vi "Actor Core.vi"(8 "error in":errorcluster, 11 "My Application":refnum<class "UI.lvclass">) -> (0 "error out":errorcluster, 3 "Actor out":refnum<class "Actor.lvclass">)   [LabVIEW 2025, in "UI.lvlib" / "UI.lvclass"]
doc: "This is Actor Core.vi, the main message handling loop for Actors. An actor usually just sits in this loop and processes messages as they arrive. Any error returned by the message Do.vi call will stop the loop, with error code 43 as the canonical signal to stop with no error sent to caller. Descendants may override that in Handle Error.vi."
uses:
  UI.lvclass
  C:/Program Files (x86)/National Instruments/LabVIEW 2025/vi.lib/ActorFramework/Actor/Actor.lvclass
  <vilib>/ActorFramework/Actor/Actor.lvclass
  Geocoding Actor/Geocoding/Country.ctl
  Geocoding Actor/Geocoding/Geocoding.lvclass
  Weather Actor/Weather/Weather.lvclass
  Geocoding Actor/Geocoding/Geocoding.lvclass/Geocoding.ctl
  Weather Actor/Weather/Weather.lvclass/Weather.ctl
  UI.lvclass/UI.ctl
  <vilib>/ActorFramework/Actor/Actor.lvclass/Actor.ctl
  <vilib>/ActorFramework/Message Enqueuer/Message Enqueuer.lvclass/Message Enqueuer.ctl
  Geocoding Actor/Geocoding Messages/Get Geo Codes Msg/Get Geo Codes Msg.lvclass/Get Geo Codes Msg.ctl
  Weather Actor/Weather Messages/Get Weather Forecast Data Msg/Get Weather Forecast Data Msg.lvclass/Get Weather Forecast Data Msg.ctl
  <vilib>/ActorFramework/Message Enqueuer/Init from Existing Queue.vi
  <vilib>/ActorFramework/Message Enqueuer/Enqueue.vi
  <vilib>/ActorFramework/Stop Msg/Stop Msg.lvclass
  C:/Program Files (x86)/National Instruments/LabVIEW 2025/vi.lib/ActorFramework/Message/Message.lvclass
  Geocoding Actor/Geocoding Messages/Get Geo Codes Msg/Get Geo Codes Msg.lvclass
  Weather Actor/Weather Messages/Get Weather Forecast Data Msg/Get Weather Forecast Data Msg.lvclass
  <vilib>/ActorFramework/Message Priority Queue/Priority Enqueue.vi
  <vilib>/ActorFramework/Message Enqueuer/Message Enqueuer.lvclass
panel:
  out "Results":T1(array[cluster])
  out "Weather Forecast Data":T2(graph)
  in  "Country":T3=enum."Germany"
  in  "City":string
  out "Table Control":string[][](table)
  in  "stop signal":bool
  in  "Stop":bool
  in  "Get City Data":bool
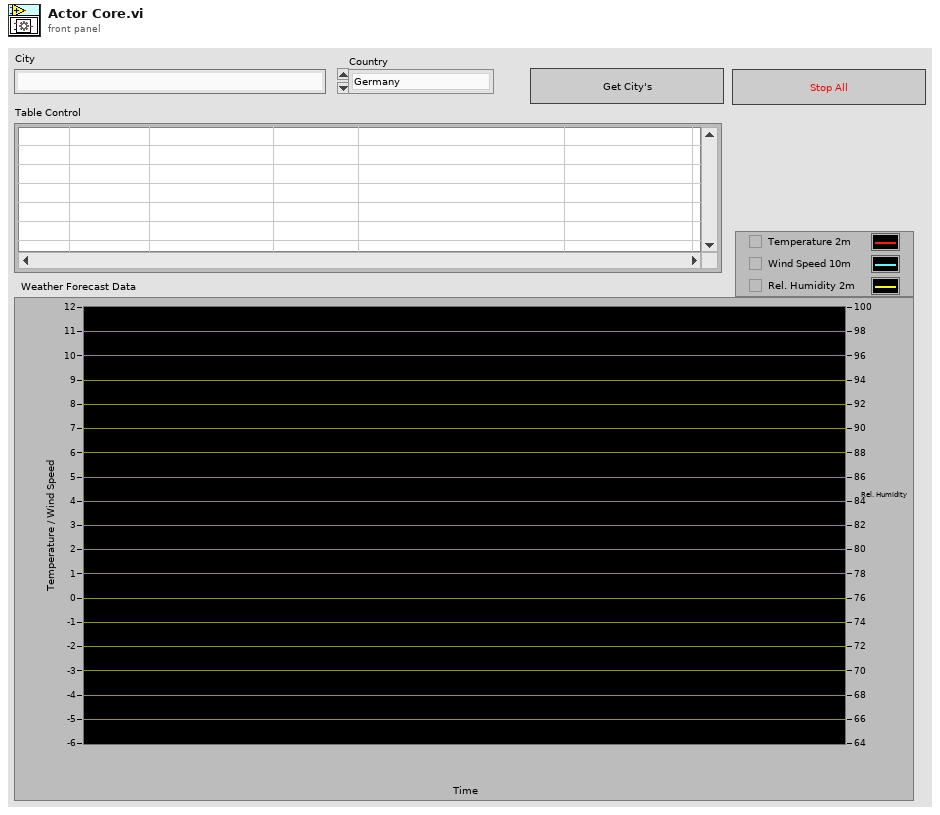
[diagram p1: front panel]
types:
  T1 = cluster{"id":i32, "name":string, "latitude":dbl, "longitude":dbl, "elevation":dbl, "feature_code":string, "country_code":string, "timezone":string, "population":i32, "postcodes":string[], "admin1":string, "admin2":string, "admin3":string, "admin4":string, "admin1_id":i32, "admin2_id":i32, "admin3_id":i32, "admin4_id":i32}[]
  T2 = cluster{timestamp[], "relative_humidity_2m":dbl[]}[]
  T3 = typedef "Geocoding Actor.lvlib/Geocoding.lvclass/Country.ctl" = enum16{"Austria", "Germany", "Switzerland"}
  T4 = typedef "LVRowAndColumnTypeDef.ctl" = cluster{"Row":i32, "Column":i32}
  T5 = cluster{"id":i32, "name":string, "latitude":dbl, "longitude":dbl, "elevation":dbl, "feature_code":string, "country_code":string, "timezone":string, "population":i32, "postcodes":string[], "admin1":string, "admin2":string, "admin3":string, "admin4":string, "admin1_id":i32, "admin2_id":i32, "admin3_id":i32, "admin4_id":i32}
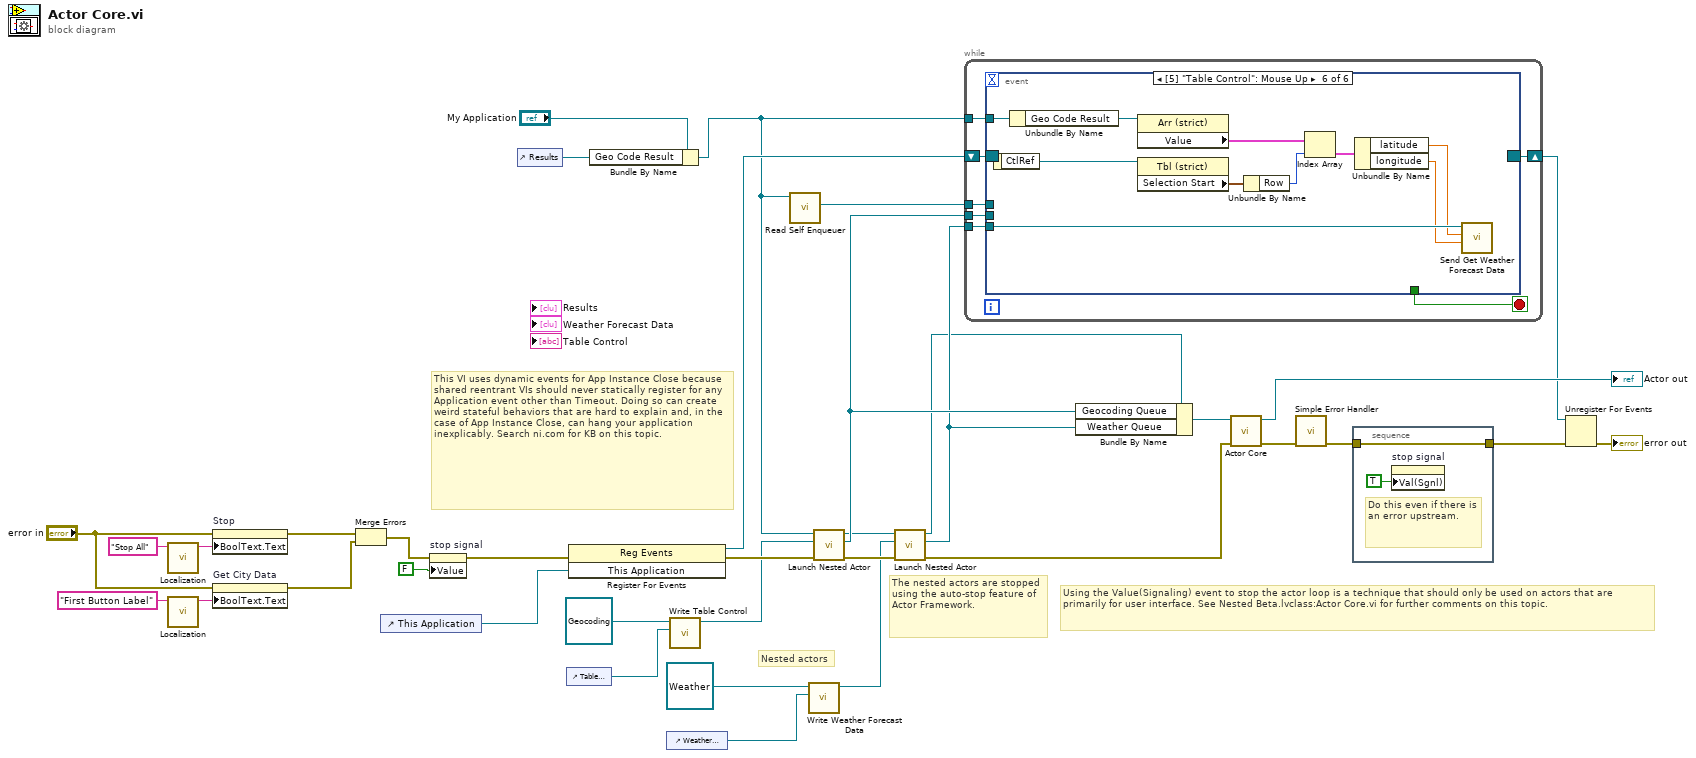
[diagram p0: block diagram]
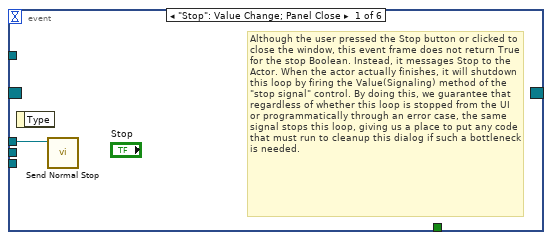
[diagram p2: hidden frame]
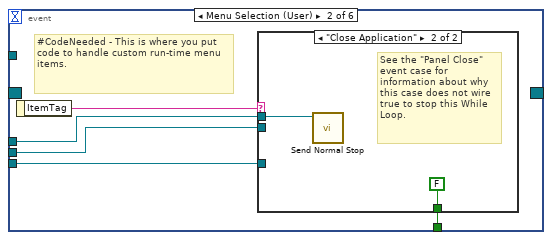
[diagram p3: hidden frame]
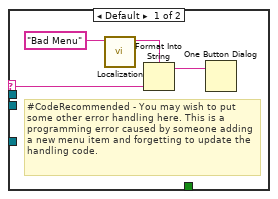
[diagram p4: hidden frame]
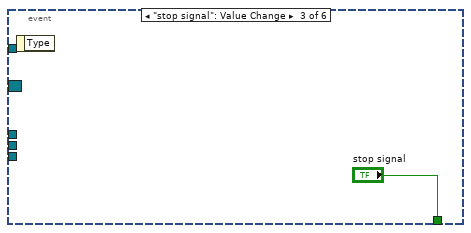
[diagram p5: hidden frame]
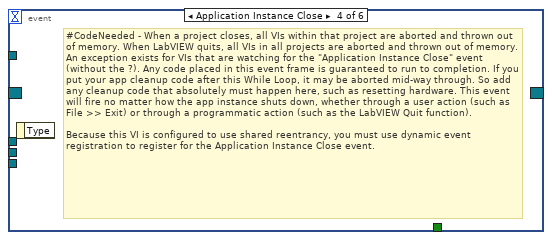
[diagram p6: hidden frame]
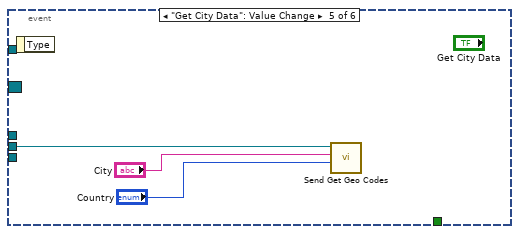
[diagram p7: hidden frame]
diagram:
  # "Nested actors"
  # "The nested actors are stopped using the auto-stop feature of Actor Framework."
  # "This VI uses dynamic events for App Instance Close because shared reentrant VIs should never statically register for any Application event other than Timeout. Doing so can create weird stateful behaviors that are hard to explain and, in the case of App Instance Close, can hang your application inexplicably. Search ni.com for KB on this topic."
  # "Using the Value(Signaling) event to stop the actor loop is a technique that should only be used on actors that are primarily for user interface. See Nested Beta.lvclass:Actor Core.vi for further comments on this topic."
  n1 = call "Localization.vi"("Unlocalized"="Stop All") -> ("Localized"=w24:string)  [unwired: 10 in]
  n2 = call "Localization.vi"("Unlocalized"="First Button Label") -> ("Localized"=w26:string)  [unwired: 10 in]
  n3 = property on="Stop" class="Bool"(error in="error in", "BoolText.Text"=w24) -> (error out=w23:errorcluster)  [unwired: 1 in, 1 out]
  n4 = property on="Get City Data" class="Bool"(error in="error in", "BoolText.Text"=w26) -> (error out=w22:errorcluster)  [unwired: 1 in, 1 out]
  n5 = Merge Errors(w23, w22) -> (w21:errorcluster)
  n6 = control-ref of="This Application"() -> (w12:refnum<vi>)
  n7 = property on="stop signal" class="Bool (strict)"(error in=w21, "Value"=FALSE ("stop")) -> (error out=w14:errorcluster)  [unwired: 1 in, 1 out]
  n8 = control-ref of="Results"() -> (w1:refnum<vi>)
  n9 = control-ref of="Table Control"() -> (w7:refnum<vi>)
  n10 = register-events(error in=w14, w12) -> (reference out=w18:refnum<event-registration>, error out=w13:errorcluster)  [unwired: 1 in]
  n11 = Bundle By Name(cluster="My Application", "Geo Code Result"=w1) -> (w2:refnum<class "UI.lvclass">)
  n12 = control-ref of="Weather Forecast Data"() -> (w4:refnum<vi>)
  n13 = call "Write Table Control.vi"("Table Control"=w7, "Geocoding in"=refnum<class "Geocoding.lvclass"> refnum ("Alpha.lvclass")) -> ("Geocoding out"=w8:refnum<class "Geocoding.lvclass">)  [unwired: 8 in, 1 out]
  n14 = call <vilib>:"Read Self Enqueuer.vi"("Actor"=w2) -> ("Self Enqueuer"=w32:refnum<class "Message Enqueuer.lvclass">)  [unwired: 10 in]
  n15 = call "Write Weather Forecast Data.vi"("Weather Forecast Data"=w4, "Weather in"=refnum<class "Weather.lvclass"> refnum ("Beta.lvclass")) -> ("Weather out"=w5:refnum<class "Weather.lvclass">)  [unwired: 8 in, 1 out]
  n16 = call <vilib>:"Launch Nested Actor.vi"("error in (no error)"=w13, "Nested Actor"=w8, "Caller Actor in"=w2) -> ("error out"=w35:errorcluster, "Nested Actor's Enqueuer"=w31:refnum<class "Message Enqueuer.lvclass">, "Caller Actor out"=w11:refnum<class "UI.lvclass">)  [unwired: 6 in]
  n17 = call <vilib>:"Launch Nested Actor.vi"("error in (no error)"=w35, "Nested Actor"=w5, "Caller Actor in"=w11) -> ("error out"=w34:errorcluster, "Nested Actor's Enqueuer"=w30:refnum<class "Message Enqueuer.lvclass">, "Caller Actor out"=w10:refnum<class "UI.lvclass">)  [unwired: 6 in]
  n18 = while {
    tunnel: w32 -> [w43]
    tunnel: w31 -> [w42]
    tunnel: w30 -> [w41]
    shift-right: [w38] -> w17
    shift-left: w18 -> [w39]
    tunnel: w2 -> [w37]
    stop <- w40 stop-if-true
    n19 = event shown="[5] \"Table Control\": Mouse Up" {
      selector: w39 -> [_ _ _ _ _ _]
      dyn-events: [_ _ _ _ _ _] -> w38
      timeout: _ -> [_ _ _ _ _ _]
      tunnel: w43 -> [w44 w46 _ _ _ _]
      tunnel: w42 -> [_ w48 _ _ w59 _]
      tunnel: w41 -> [_ w47 _ _ _ w67]
      tunnel: [_ w45 "stop signal" _ _ _] -> w40
      tunnel: w37 -> [_ _ _ _ _ w64]
      event "Stop": Value Change; Panel Close {
        # "Although the user pressed the Stop button or clicked to close the window, this event frame does not return True for the stop Boolean. Instead, it messages Stop to the Actor. When the actor actually finishes, it will shutdown this loop by firing the Value(Signaling) method of the \"stop signal\" control. By doing this, we guarantee that regardless of whether this loop is stopped from the UI or programmatically through an error case, the same signal stops this loop, giving us a place to put any code that must run to cleanup this dialog if such a bottleneck is needed."
        n20 = event-data() -> ()  [unwired: 1 in, 1 out]
        n21 = call <vilib>:"Send Normal Stop.vi"("Message Enqueuer"=w44) -> ()  [unwired: 10 in, 1 out]
      }
      event Menu Selection (User) {
        # "#CodeNeeded - This is where you put code to handle custom run-time menu items."
        n22 = event-data() -> ("ItemTag"=w49:string)  [unwired: 1 in]
        n23 = case shown="\"Close Application\"" w49 {
          selector: w49 -> [w51 _]
          tunnel: w48 -> [_ _]
          tunnel: w47 -> [_ _]
          tunnel: w46 -> [_ w54]
          tunnel: [_ FALSE] -> w45
          frame Default {
            # "#CodeRecommended - You may wish to put some other error handling here. This is a programming error caused by someone adding a new menu item and forgetting to update the handling code."
            n24 = call "Localization.vi"("Unlocalized"="Bad Menu") -> ("Localized"=w52:string)  [unwired: 10 in]
            n25 = Format Into String(format string=w52, w51) -> (resulting string=w50:string)  [unwired: 2 in, 1 out]
            n26 = One Button Dialog(message=w50) -> ()  [unwired: 1 in, 1 out]
          }
          frame "Close Application" {
            # "See the \"Panel Close\" event case for information about why this case does not wire true to stop this While Loop."
            n27 = call <vilib>:"Send Normal Stop.vi"("Message Enqueuer"=w54) -> ()  [unwired: 10 in, 1 out]
          }
        }
      }
      event "stop signal": Value Change {
        n28 = event-data() -> ()  [unwired: 1 in, 1 out]
      }
      event Application Instance Close {
        # "#CodeNeeded - When a project closes, all VIs within that project are aborted and thrown out of memory. When LabVIEW quits, all VIs in all projects are aborted and thrown out of memory. An exception exists for VIs that are watching for the \"Application Instance Close\" event (without the ?). Any code placed in this event frame is guaranteed to run to completion. If you put your app cleanup code after this While Loop, it may be aborted mid-way through. So add any cleanup code that absolutely must happen here, such as resetting hardware. This event will fire no matter how the app instance shuts down, whether through a user action (such as File >> Exit) or through a programmatic action (such as the LabVIEW Quit function).\n\nBecause this VI is configured to use shared reentrancy, you must use dynamic event registration to register for the Application Instance Close event."
        n29 = event-data() -> ()  [unwired: 1 in, 1 out]
      }
      event "Get City Data": Value Change {
        n30 = event-data() -> ()  [unwired: 1 in, 1 out]
        n31 = call "Send Get Geo Codes.vi"("Country"="Country", "City Name"="City", "Message Enqueuer"=w59) -> ()  [unwired: 7 in, 2 out]
      }
      event "Table Control": Mouse Up {
        n32 = event-data() -> ("CtlRef"=w60:refnum<vi>)  [unwired: 1 in]
        n33 = Unbundle By Name(w64) -> ("Geo Code Result"=w63:refnum<vi>)
        n34 = property class="Arr (strict)"(reference=w63) -> ("Value"=w69:T1)  [unwired: 1 in, 2 out]
        n35 = property class="Tbl (strict)"(reference=w60) -> ("Selection Start"=w62:T4)  [unwired: 1 in, 2 out]
        n36 = Unbundle By Name(w62) -> ("Row"=w61:i32)
        n37 = Index Array(array=w69, index=w61) -> (element=w68:T5)
        n38 = Unbundle By Name(w68) -> ("latitude"=w65:dbl, "longitude"=w66:dbl)
        n39 = call "Send Get Weather Forecast Data.vi"("Longitude"=w66, "Latitude"=w65, "Message Enqueuer"=w67) -> ()  [unwired: 7 in, 2 out]
      }
    }
  }
  n40 = Bundle By Name(cluster=w10, "Geocoding Queue"=w31, "Weather Queue"=w30) -> (w33:refnum<class "UI.lvclass">)
  n41 = call-parent "Actor Core.vi"("error in"=w34, "Actor in"=w33) -> ("error out"=w20:errorcluster, "Actor out"=→"Actor out":refnum<class "Actor.lvclass">)  [unwired: 8 in]
  n42 = call <vilib>:"Simple Error Handler.vi"("error in (no error)"=w20) -> ("error out"=w19:errorcluster)  [unwired: 4 in, 4 out]
  n43 = stacked-sequence {
    tunnel: [w70] -> w16
    tunnel: w19 -> [w70]
    frame #0 {
      # "Do this even if there is an error upstream."
      n44 = property on="stop signal" class="Bool (strict)"("Val(Sgnl)"=TRUE ("stop")) -> ()  [unwired: 2 in, 2 out]
    }
  }
  n45 = Unregister For Events(event registration refnum=w17, error in=w16) -> (error out=→"error out":errorcluster)
